vi "Memory Cell to vec3d.vi"(10 "Memory Cell":T1={"type"=enum."vector", "x"=0.0, "y"=0.0, "z"=0.0, "w"=0.0}) -> (2 "Vec3d out":refnum<class "Vec3d.lvclass">)   [LabVIEW 2024]
uses:
  Type Definitions/Memory Cell.ctl
  Type Definitions/Memory Cell Type Enum.ctl
  Shared Components/Vec3d Class/Vec3d.lvclass
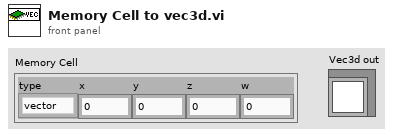
[diagram p1: front panel]
types:
  T1 = typedef "Memory Cell.ctl" = cluster{"type":T2, "x":dbl, "y":dbl, "z":dbl, "w":dbl}
  T2 = typedef "Memory Cell Type Enum.ctl" = enum16{"integer", "float", "vector", "rotation"}
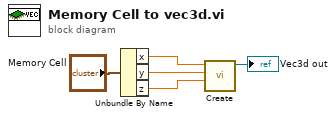
[diagram p0: block diagram]
diagram:
  n1 = Unbundle By Name("Memory Cell") -> ("x"=w4:dbl, "y"=w3:dbl, "z"=w2:dbl)
  n2 = call "Create.vi"("Z"=w2, "Y"=w3, "X"=w4) -> ("Vec3d Class out"=→"Vec3d out":refnum<class "Vec3d.lvclass">)  [unwired: 7 in, 1 out]
